vi "SubVI -  inline.vi"(1 "Array in":dbl[](array[numeric])) -> (0 "Array":dbl[](array[numeric]))   [LabVIEW 2025]
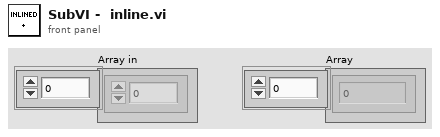
[diagram p1: front panel]
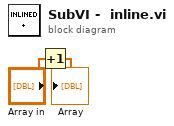
[diagram p0: block diagram]
diagram:
  n1 = Increment(x="Array in") -> (x+1=→"Array":dbl[])
